vi "ATSh_SetLED.vi"(6 "state":bool, 7 "Handle":u32) -> (0 "Return_Code":u32)   [LabVIEW 2010]
doc: "_____AlazarTech, Scope_____\n\nTurn ON or OFF the LED found on the devices panel.\n\nInput:\n\"Handle\" = handle of the board\n\"State\" = On or Off\n\nOutput:\n\"Return_Code\"= 512"
uses:
  ATSApi.dll
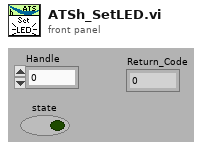
[diagram p1: front panel]
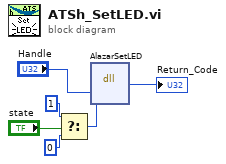
[diagram p0: block diagram]
diagram:
  n1 = Select(t=u32 1, s="state", f=u32 0) -> (s? t:f=w3:u32)
  n2 = dll-call lib="ATSApi.dll" fn="AlazarSetLED"("Handle"="Handle", "state"=w3) -> (→"Return_Code":u32)  [unwired: 5 in, 2 out]
